vi "ExPlugin_COMMAND.vi"(6 "WEB in":T2={"Services Page"="", "Login"="", "Password"="", "Cookie file"=path "", "Timeout"=0.0, "Verify server"=TRUE, "Client handle"=refnum}, 7 "REST API in":T1, 8 "error in (no error)":errorcluster, 9 "command":string, 10 "name":string, 11 "Mode out":enum16{"get", "set", "close", "Init", "Check"}(ring)) -> (0 "error out":errorcluster, 2 "Response":string, 4 "WEB out":T2={"Services Page"="", "Login"="", "Password"="", "Cookie file"=path "", "Timeout"=0.0, "Verify server"=TRUE, "Client handle"=refnum}, 5 "REST API out":T1)   [LabVIEW 2018]
uses:
  Llb/HTTP.llb/WEB info.ctl
  <vilib>/httpClient/ClientHandle.ctl
  Llb/HTTP.llb/REST API.ctl
  Llb/HTTP.llb/WEB method.ctl
  Llb/HTTP.llb/HTTP.lvlib
  <vilib>/httpClient/LabVIEWHTTPClient.lvlib
  Llb/HTTP.llb/REST API.lvlib
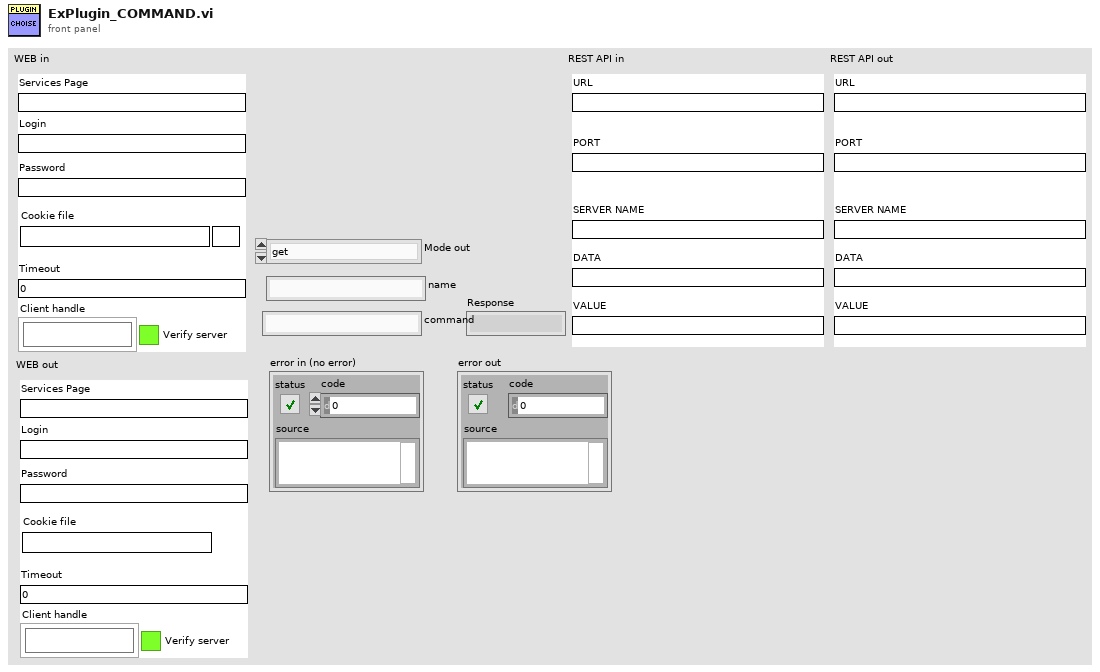
[diagram p1: front panel]
types:
  T1 = typedef "REST API.lvlib/REST API.ctl" = cluster{"URL":string, "PORT":string, "SERVER NAME":string, "DATA":string, "VALUE":string}
  T2 = typedef "HTTP.lvlib/WEB info.ctl" = cluster{"Services Page":string, "Login":string, "Password":string, "Cookie file":path, "Timeout":dbl, "Verify server":bool, "Client handle":T3}
  T3 = typedef "LabVIEWHTTPClient.lvlib/ClientHandle.ctl" = refnum<k1>
  T4 = typedef "HTTP.lvlib/WEB method.ctl" = string
  T5 = typedef "HTTP.lvlib/Error out.ctl" = errorcluster
  T6 = typedef "HTTP.lvlib/WEB response.ctl" = cluster{"Header":string, "Body":string}
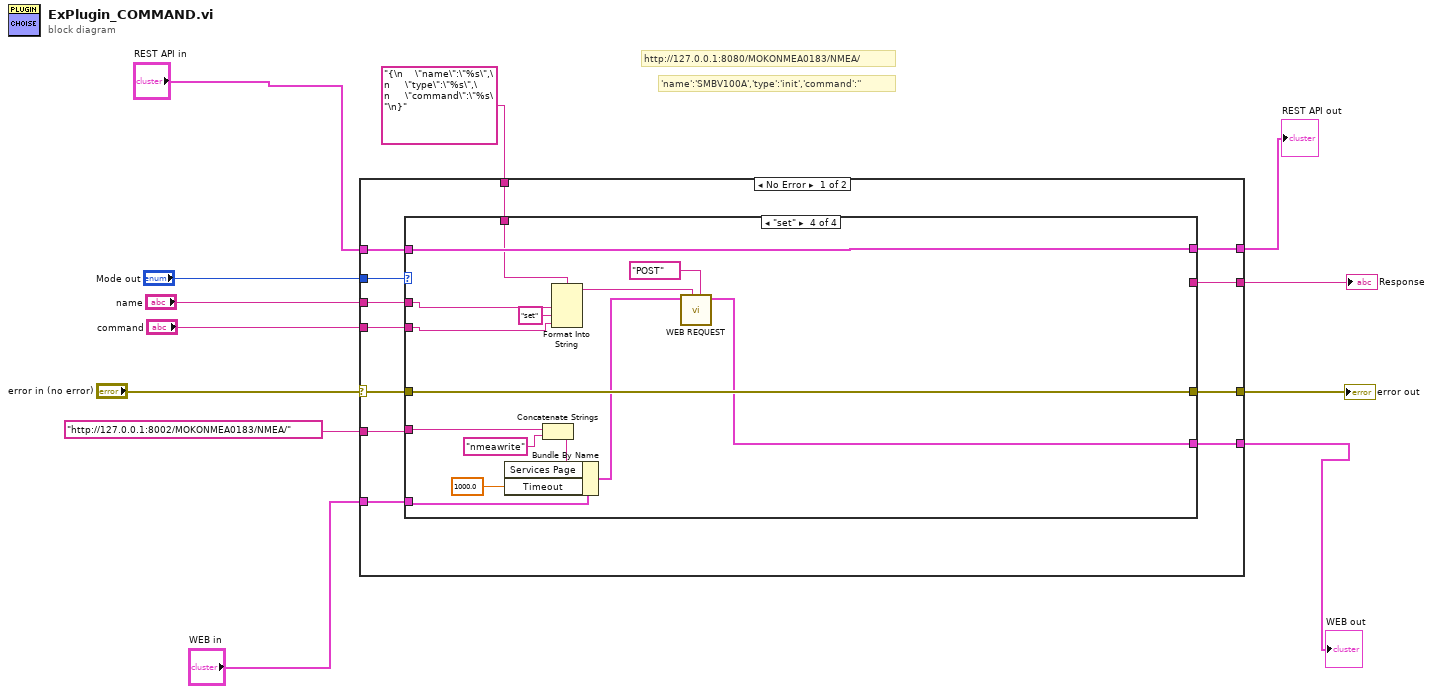
[diagram p0: block diagram]
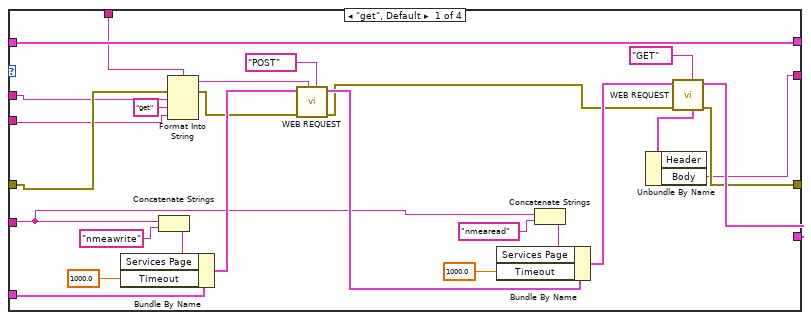
[diagram p2: hidden frame]
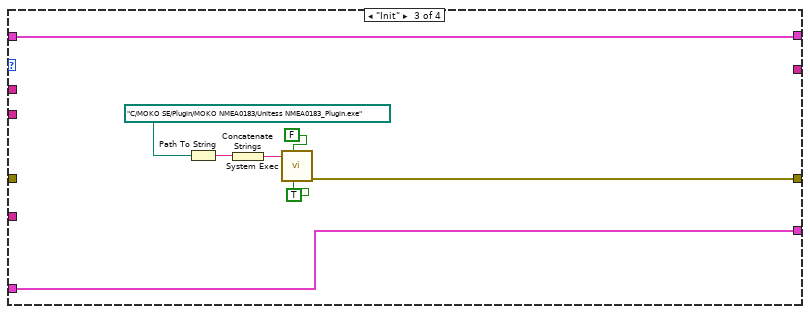
[diagram p4: hidden frame]
diagram:
  # "http://127.0.0.1:8080/MOKONMEA0183/NMEA/"
  # "'name':'SMBV100A','type':'init','command':''"
  n1 = case shown="No Error" "error in (no error)" {
    selector: "error in (no error)" -> [w23 w78]
    tunnel: [w22 w78] -> w11
    tunnel: [w19 _] -> w1
    tunnel: "Mode out" -> [w24 _]
    tunnel: "name" -> [w21 _]
    tunnel: "command" -> [w20 _]
    tunnel: [w18 w77] -> w7
    tunnel: "WEB in" -> [w17 w77]
    tunnel: [w16 w76] -> w5
    tunnel: "REST API in" -> [w15 w76]
    tunnel: "http://127.0.0.1:8002/MOKONMEA0183/NMEA/" -> [w14 _]
    tunnel: "{\n    \"name\":\"%s\",\n     \"type\":\"%s\",\n     \"command\":\"%s\"\n}" -> [w13 _]
    frame No Error {
      n2 = case shown="\"set\"" w24 {
        tunnel: w23 -> [w34 _ _ w75]
        tunnel: [w32 _ w55 w75] -> w22
        tunnel: w21 -> [w29 _ _ w71]
        tunnel: w20 -> [w28 _ _ w69]
        tunnel: [w25 _ _ _] -> w19
        tunnel: [w37 w52 w54 w73] -> w18
        tunnel: w17 -> [w30 w52 w54 w66]
        tunnel: [w50 w51 w53 w74] -> w16
        tunnel: w15 -> [w50 w51 w53 w74]
        tunnel: w14 -> [w35 _ _ w64]
        tunnel: w13 -> [w31 _ _ w61]
        frame "get", Default {
          n3 = Concatenate Strings(w35, "nmeawrite" ("string")) -> (w45:string)
          n4 = Bundle By Name(cluster=w30, "Services Page"=w45, "Timeout"=1000.0) -> (w43:T2)
          n5 = Format Into String(format string=w31, error in=w34, w29, "get" ("input 2"), w28) -> (resulting string=w47:string, error out=w33:errorcluster)  [unwired: 1 in]
          n6 = call "WEB REQUEST.vi"("WEB method"=T4 "POST", "Data"=w47, "error in"=w33, "WEB in"=w43) -> ("error out"=w27:T5, "WEB out"=w36:T2)  [unwired: 5 in, 1 out]
          n7 = Concatenate Strings(w35, "nmearead" ("string")) -> (w40:string)
          n8 = Bundle By Name(cluster=w36, "Services Page"=w40, "Timeout"=1000.0) -> (w38:T2)
          n9 = call "WEB REQUEST.vi"("WEB method"=T4 "GET", "error in"=w27, "WEB in"=w38) -> ("error out"=w32:T5, "WEB out"=w37:T2, "WEB response"=w26:T6)  [unwired: 6 in]
          n10 = Unbundle By Name(w26) -> ("Body"=w25:string)  [unwired: 1 out]
        }
        frame "close" {
        }
        frame "Init" {
          n11 = Path To String(path=path "C:/MOKO SE/Plugin/MOKO NMEA0183/Unitess NMEA0183_Plugin.exe" ("File Path Control 2")) -> (string=w59:string)
          n12 = Concatenate Strings(w59) -> (w60:string)
          n13 = call <vilib>:"System Exec.vi"("run minimized? (F)"=TRUE, "wait until completion? (T)"=FALSE, "command line"=w60) -> ("error out"=w55:errorcluster)  [unwired: 3 in, 5 out]
        }
        frame "set" {
          n14 = Concatenate Strings(w64, "nmeawrite" ("string")) -> (w65:string)
          n15 = Bundle By Name(cluster=w66, "Services Page"=w65, "Timeout"=1000.0) -> (w62:T2)
          n16 = Format Into String(format string=w61, w71, "set" ("input 2"), w69) -> (resulting string=w68:string)  [unwired: 2 in, 1 out]
          n17 = call "WEB REQUEST.vi"("WEB method"=T4 "POST", "Data"=w68, "WEB in"=w62) -> ("WEB out"=w73:T2)  [unwired: 6 in, 2 out]
        }
      }
    }
    frame Error {
    }
  }
  "Response" <- w1
  "error out" <- w11
  "WEB out" <- w7
  "REST API out" <- w5
